vi "sub_gridmap_calc-config.vi"   [LabVIEW 2019]
uses:
  Ctrl/cmd_common.ctl
types:
  T1 = typedef "cmd_common.ctl" = enum16{"read", "write"}
  T2 = typedef "NI_Matrix.lvlib/RealMatrix.ctl" = dbl[][]
  T3 = cluster{"ox":T2, "oy":T2, "x_est":T2, "x_true":T2, "u":T2, "z":T2, "PEst":T2, "min x":dbl, "min y":dbl, "max x":dbl, "max y":dbl, "yw":i32, "xw":i32}
  T4 = cluster{"resolution":dbl, "EXTEND_AREA":dbl, "MAX_RANGE":dbl, "NP":u32, "NTh":u32, "Q":T2, "R":T2, "Q_sim":T2, "R_sim":T2, "rf_id":cluster{"x":dbl, "y":dbl}[]}
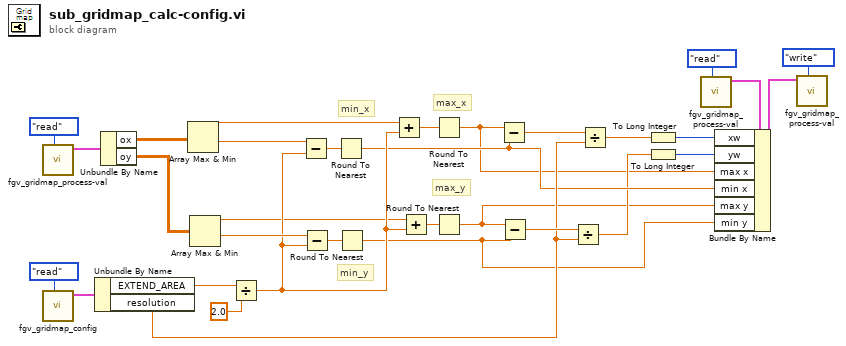
[diagram p0: block diagram]
diagram:
  # "max_y"
  # "max_x"
  # "min_y"
  # "min_x"
  n1 = call "fgv_gridmap_process-val.vi"("cmd"=cmd_common."read") -> ("p-val out"=w30:T3)  [unwired: 10 in]
  n2 = call "fgv_gridmap_config.vi"("cmd"=cmd_common."read") -> ("pf-val out"=w27:T4)  [unwired: 10 in]
  n3 = Unbundle By Name(w27) -> ("EXTEND_AREA"=w26:dbl, "resolution"=w8:dbl)
  n4 = Unbundle By Name(w30) -> ("ox"=w29:T2, "oy"=w28:T2)
  n5 = Array Max & Min(array=w29) -> (max value=w14:dbl, min value=w20:dbl)  [unwired: 2 out]
  n6 = Array Max & Min(array=w28) -> (max value=w12:dbl, min value=w15:dbl)  [unwired: 2 out]
  n7 = Divide(x=w26, y=2.0) -> (x/y=w13:dbl)
  n8 = Subtract(x=w20, y=w13) -> (x-y=w17:dbl)
  n9 = Subtract(x=w15, y=w13) -> (x-y=w16:dbl)
  n10 = Round To Nearest(number=w17) -> (nearest integer value=w7:dbl)
  n11 = Round To Nearest(number=w16) -> (nearest integer value=w4:dbl)
  n12 = Add(x=w14, y=w13) -> (x+y=w6:dbl)
  n13 = Add(x=w12, y=w13) -> (x+y=w5:dbl)
  n14 = Round To Nearest(number=w6) -> (nearest integer value=w2:dbl)
  n15 = Round To Nearest(number=w5) -> (nearest integer value=w1:dbl)
  n16 = Subtract(x=w2, y=w7) -> (x-y=w11:dbl)
  n17 = Subtract(x=w1, y=w4) -> (x-y=w9:dbl)
  n18 = Divide(x=w9, y=w8) -> (x/y=w3:dbl)
  n19 = Divide(x=w11, y=w8) -> (x/y=w10:dbl)
  n20 = To Long Integer(number=w10) -> (32bit integer=w19:i32)
  n21 = To Long Integer(number=w3) -> (32bit integer=w18:i32)
  n22 = call "fgv_gridmap_process-val.vi"("cmd"=cmd_common."read") -> ("p-val out"=w22:T3)  [unwired: 10 in]
  n23 = Bundle By Name(cluster=w22, "xw"=w19, "yw"=w18, "max x"=w2, "min x"=w7, "max y"=w1, "min y"=w4) -> (w21:T3)
  n24 = call "fgv_gridmap_process-val.vi"("cmd"=cmd_common."write", "p-val"=w21) -> ()  [unwired: 9 in, 1 out]
